vi "Config Line Filter and Zero Cross.vi"(0 "VISA resource name":refnum<visa-resource-name>, 1 "Scaling (F: OFF)":bool, 5 "Element (0: ALL)":u16(ring) items=["All", "Element 1", "Element 2", "Element 3", "Element 4"], 7 "Line Filter (0: OFF)":u16(ring) items=["OFF", "500Hz", "20kHz", "1MHz"], 9 "Zero Cross Filter (0: OFF)":u16(ring) items=["OFF", "500Hz", "20kHz"], 11 "error in (no error)":errorcluster, 12 "PT Ratio (1.00)":dbl=1.0 min=0.0001 max=99999.9999 step=0.0001 format="%.4f", 13 "CT Ratio (1.00)":dbl=1.0 min=0.0001 max=99999.9999 step=0.0001 format="%.4f", 14 "Scaling Factor (1.00)":dbl=1.0 min=0.0001 max=99999.9999 step=0.0001 format="%.4f") -> (4 "VISA resource name out":refnum<visa-resource-name>, 15 "error out":errorcluster)   [LabVIEW 2014, in "Yokogawa.lvlib" / "Yokogawa PZ4000.lvlib"]
doc: "This VI sends the Line filter and ZeroCross Configure command to the PZ4000 series.\nConfigure Control Functions are Line Filter ,Zero Cross Filter, Scaling, PT Ratio, CT Ratio, Scaling Factor."
uses:
  Yokogawa PZ4000.lvlib
panel:
  # "ON\nOFF"
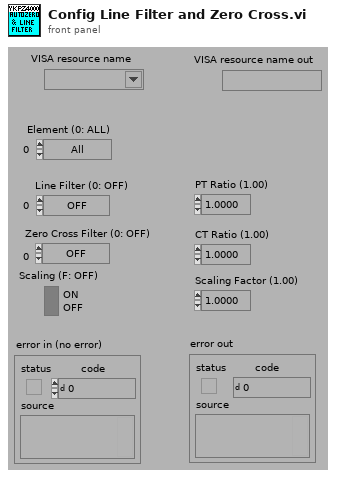
[diagram p1: front panel]
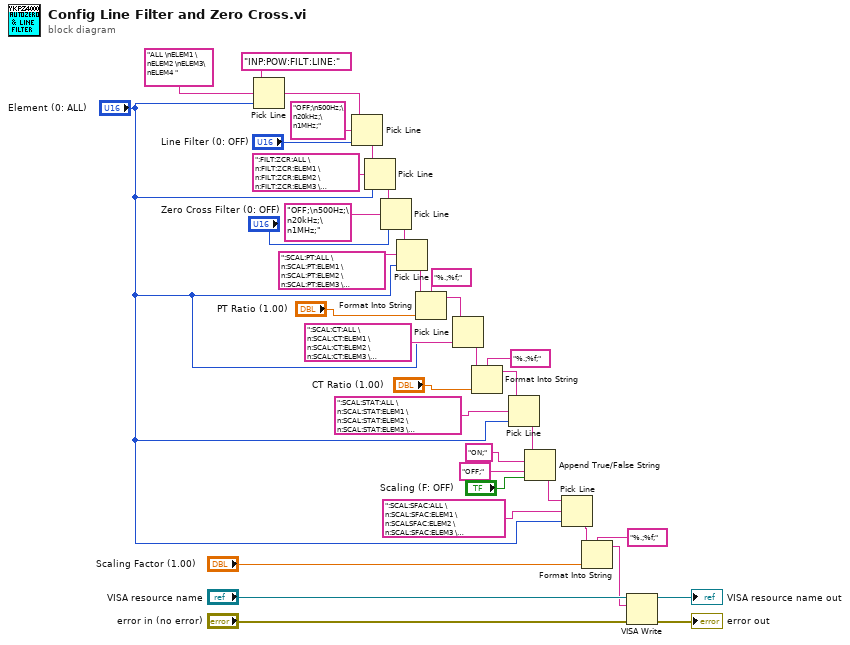
[diagram p0: block diagram]
diagram:
  n1 = Pick Line(string ("")="INP:POW:FILT:LINE:", multi-line string="ALL \nELEM1 \nELEM2 \nELEM3\nELEM4 ", line index="Element (0: ALL)") -> (output string=w31:string)
  n2 = Pick Line(string ("")=w31, multi-line string="OFF;\n500Hz;\n20kHz;\n1MHz;", line index="Line Filter (0: OFF)") -> (output string=w28:string)
  n3 = Pick Line(string ("")=w28, multi-line string=":FILT:ZCR:ALL \n:FILT:ZCR:ELEM1 \n:FILT:ZCR:ELEM2 \n:FILT:ZCR:ELEM3 \n:FILT:ZCR:ELEM4 ", line index="Element (0: ALL)") -> (output string=w26:string)
  n4 = Pick Line(string ("")=w26, multi-line string="OFF;\n500Hz;\n20kHz;\n1MHz;", line index="Zero Cross Filter (0: OFF)") -> (output string=w18:string)
  n5 = Pick Line(string ("")=w18, multi-line string=":SCAL:PT:ALL \n:SCAL:PT:ELEM1 \n:SCAL:PT:ELEM2 \n:SCAL:PT:ELEM3 \n:SCAL:PT::ELEM4 ", line index="Element (0: ALL)") -> (output string=w15:string)
  n6 = Format Into String(format string="%.;%f;", initial string=w15, "PT Ratio (1.00)") -> (resulting string=w12:string)  [unwired: 1 in, 1 out]
  n7 = Pick Line(string ("")=w12, multi-line string=":SCAL:CT:ALL \n:SCAL:CT:ELEM1 \n:SCAL:CT:ELEM2 \n:SCAL:CT:ELEM3 \n:SCAL:CT::ELEM4 ", line index="Element (0: ALL)") -> (output string=w11:string)
  n8 = Format Into String(format string="%.;%f;", initial string=w11, "CT Ratio (1.00)") -> (resulting string=w1:string)  [unwired: 1 in, 1 out]
  n9 = Pick Line(string ("")=w1, multi-line string=":SCAL:STAT:ALL \n:SCAL:STAT:ELEM1 \n:SCAL:STAT:ELEM2 \n:SCAL:STAT:ELEM3 \n:SCAL:STAT::ELEM4 ", line index="Element (0: ALL)") -> (output string=w6:string)
  n10 = Append True/False String(1:"Scaling (F: OFF)", 2:"OFF;", 3:"ON;", 4:w6) -> (0:w5:string)
  n11 = Pick Line(string ("")=w5, multi-line string=":SCAL:SFAC:ALL \n:SCAL:SFAC:ELEM1 \n:SCALSFAC:ELEM2 \n:SCAL:SFAC:ELEM3 \n:SCAL:SFAC::ELEM4 ", line index="Element (0: ALL)") -> (output string=w3:string)
  n12 = Format Into String(format string="%.;%f;", initial string=w3, "Scaling Factor (1.00)") -> (resulting string=w2:string)  [unwired: 1 in, 1 out]
  n13 = VISA Write(VISA resource name="VISA resource name", write buffer=w2, error in (no error)="error in (no error)") -> (VISA resource name out=→"VISA resource name out":refnum<visa-resource-name>, error out=→"error out":errorcluster)  [unwired: 1 out]
